vi "TracePoint_CreateDataEvent.vi"(6 "Ir Data Event":T9, 8 "error in (no error)":errorcluster, 9 "data":T12, 10 "data event":T1, 11 "Qbus":refnum<class "Qbus.lvclass">) -> (0 "error out":errorcluster)   [LabVIEW 2017, in "IrDataEventCreator.lvlib"]
uses:
  <vilib>/addons/InsightCM/Devices/Shared/Ir/IrDataEventCreator/IrDataEventCreator.lvlib
  <vilib>/addons/Qbus/Qbus.lvclass
  <vilib>/addons/InsightCM/Devices/Shared/Common/DataFlow/controls/Data.ctl
  <vilib>/addons/InsightCM/Utilities/DataAccessors/controls/wfmSGL_DVR.ctl
  <vilib>/addons/PointValueMap/controls/PointMap.ctl
  <vilib>/addons/InsightCM/Devices/Shared/Common/DataFlow/controls/Type.ctl
  <vilib>/addons/InsightCM/Devices/Shared/Ir/IrDataEventCreator/controls/IrDataEvent.ctl
  <vilib>/addons/InsightCM/Devices/Shared/Common/DataEvent/controls/EventReference.ctl
  <vilib>/addons/InsightCM/Devices/Shared/Common/DataEvent/controls/Event.ctl
  <vilib>/addons/InsightCM/MessageBus/Base/controls/DataEvent.ctl
  <vilib>/addons/InsightCM/MessageBus/Base/controls/KeyValuePair.ctl
  <vilib>/addons/InsightCM/Devices/Shared/Common/DataEvent/controls/DataSet.ctl
  <vilib>/addons/InsightCM/MessageBus/Base/controls/DataSetMetadata.ctl
  <vilib>/addons/InsightCM/MessageBus/Base/controls/TrendPoint.ctl
  <vilib>/addons/InsightCM/MessageBus/Base/controls/TrendAlarmUpdate.ctl
  <vilib>/addons/InsightCM/MessageBus/Base/controls/TrendAlarmTransition.ctl
  <vilib>/addons/TraceLogger/TraceLogger.lvlib
  <vilib>/addons/InsightCM/Devices/Shared/Common/DataEvent/DataEvent.lvlib
  <vilib>/addons/PointValueMap/PointValueMap.lvlib
  <vilib>/addons/InsightCM/Devices/Shared/Common/DataFlow/DataFlow.lvlib
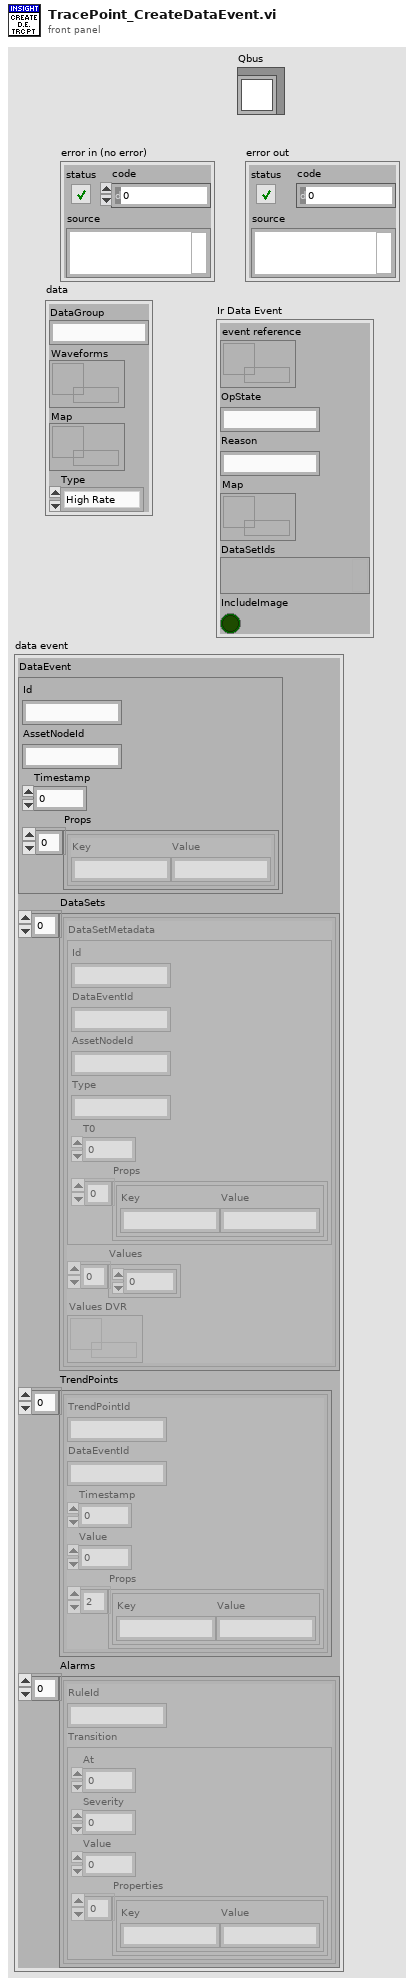
[diagram p1: front panel]
types:
  T1 = typedef "DataEvent.lvlib/Event.ctl" = cluster{"DataEvent":T2, "DataSets":T4[], "TrendPoints":T6[], "Alarms":T7[]}
  T2 = typedef "DataEvent.ctl" = cluster{"Id":string, "AssetNodeId":string, "Timestamp":i64, "Props":T3[]}
  T3 = typedef "KeyValuePair.ctl" = cluster{"Key":string, "Value":string}
  T4 = typedef "DataEvent.lvlib/DataSet.ctl" = cluster{"DataSetMetadata":T5, "Values":sgl[], "Values DVR":refnum<data-value>}
  T5 = typedef "DataSetMetadata.ctl" = cluster{"Id":string, "DataEventId":string, "AssetNodeId":string, "Type":string, "T0":i64, "Props":T3[]}
  T6 = typedef "TrendPoint.ctl" = cluster{"TrendPointId":string, "DataEventId":string, "Timestamp":i64, "Value":dbl, "Props":T3[]}
  T7 = typedef "TrendAlarmUpdate.ctl" = cluster{"RuleId":string, "Transition":T8}
  T8 = typedef "TrendAlarmTransition.ctl" = cluster{"At":i64, "Severity":i32, "Value":dbl, "Properties":T3[]}
  T9 = typedef "IrDataEventCreator.lvlib/IrDataEvent.ctl" = cluster{"event reference":T10, "OpState":string, "Reason":string, "Map":T11, "DataSetIds":variant, "IncludeImage":bool}
  T10 = typedef "DataEvent.lvlib/EventReference.ctl" = refnum<data-value>
  T11 = typedef "PointValueMap.lvlib/PointMap.ctl" = refnum<data-value>
  T12 = typedef "DataFlow.lvlib/Data.ctl" = cluster{"DataGroup":string, "Waveforms":T13, "Map":T11, "Type":T14}
  T13 = typedef "wfmSGL_DVR.ctl" = refnum<data-value>
  T14 = typedef "DataFlow.lvlib/Type.ctl" = enum16{"High Rate", "Low Rate", "Burst Mode"}
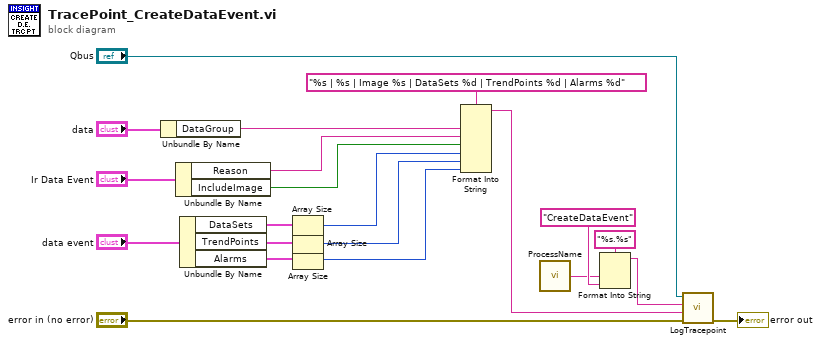
[diagram p0: block diagram]
diagram:
  n1 = Unbundle By Name("data") -> ("DataGroup"=w11:string)
  n2 = Unbundle By Name("Ir Data Event") -> ("Reason"=w15:string, "IncludeImage"=w1:bool)
  n3 = Unbundle By Name("data event") -> ("DataSets"=w7:T4[], "TrendPoints"=w6:T6[], "Alarms"=w5:T7[])
  n4 = Array Size(array=w7) -> (size(s)=w4:i32)
  n5 = Array Size(array=w6) -> (size(s)=w3:i32)
  n6 = Array Size(array=w5) -> (size(s)=w2:i32)
  n7 = Format Into String(format string="%s | %s | Image %s | DataSets %d | TrendPoints %d | Alarms %d", w11, w15, w1, w4, w3, w2) -> (resulting string=w14:string)  [unwired: 2 in, 1 out]
  n8 = call <vilib>:"ProcessName.vi"() -> ("process name"=w10:string)  [unwired: 5 in]
  n9 = Format Into String(format string="%s.%s", w10, "CreateDataEvent" ("tracepoint")) -> (resulting string=w17:string)  [unwired: 2 in, 1 out]
  n10 = call <vilib>:"LogTracepoint.vi"("error in (no error)"="error in (no error)", "log string"=w14, "tracepoint"=w17, "qbus in"="Qbus") -> ("error out"=→"error out":errorcluster)  [unwired: 6 in, 1 out]
